vi "onCreateListener.vi"(6 "timeout (ms)":i32=100, 8 "error in (no error)":errorcluster, 10 "Configuration":refnum<class "Connection.Collection.lvclass">) -> (0 "error out":errorcluster, 3 "Listener":refnum<class "Connection.lvclass">)   [LabVIEW 2013, in "Connection_GOSPL.lvlib" / "Connection.Collection.lvclass"]
uses:
  Connection.Collection.lvclass
  Connection/Connection.lvclass
  Connection.Collection.lvclass/Connection.Collection.ctl
  Connection/Connection.lvclass/Connection.ctl
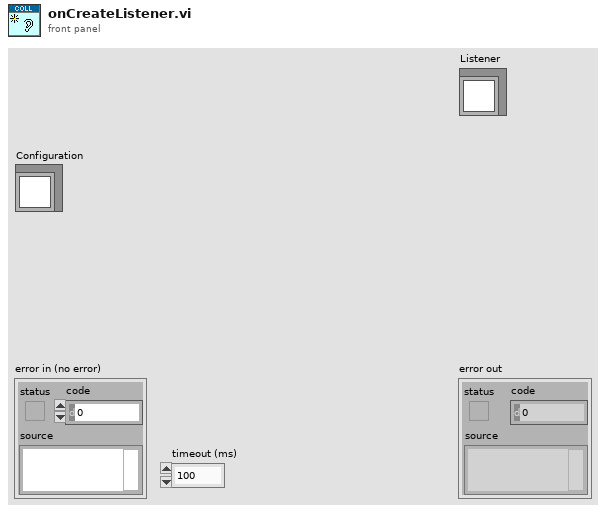
[diagram p1: front panel]
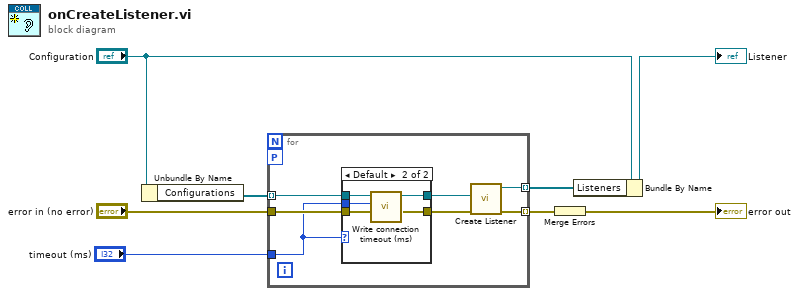
[diagram p0: block diagram]
diagram:
  n1 = Unbundle By Name("Configuration") -> ("Configurations"=w4:refnum<class "Connection.lvclass">[])
  n2 = for {
    tunnel: "error in (no error)" -> [w11]
    tunnel: [w14] -> w6 mode=indexing
    tunnel: w4 -> [w13] mode=indexing
    tunnel: [w15] -> w3 mode=indexing
    workers-P: _ -> [_]
    tunnel: "timeout (ms)" -> [w9]
    n3 = case shown="Default" w9 {
      tunnel: w13 -> [w17 w22]
      tunnel: [w17 w21] -> w12
      tunnel: w11 -> [w16 w20]
      tunnel: [w16 w19] -> w10
      tunnel: w9 -> [_ w18]
      frame ..-1 {
      }
      frame Default {
        n4 = call "Write connection timeout (ms).vi"("error in (no error)"=w20, "connection timeout (ms)"=w18, "Connection in"=w22) -> ("error out"=w19:errorcluster, "Connection out"=w21:refnum<class "Connection.lvclass">)  [unwired: 7 in]
      }
    }
    n5 = call "Create Listener.vi"("error in (no error)"=w10, "Connection Configuration"=w12) -> ("error out"=w14:errorcluster, "Listener"=w15:refnum<class "Connection.lvclass">)  [unwired: 8 in]
  }
  n6 = Merge Errors(w6) -> (→"error out":errorcluster)
  n7 = Bundle By Name(cluster="Configuration", "Listeners"=w3) -> (→"Listener":refnum<class "Connection.Collection.lvclass">)
